vi "Test Gripper.vi"() -> ()   [LabVIEW 2018]
uses:
  <vilib>/Rock Robotics/SystemInterfaces/DIO/FPGA_DIOChannel.ctl
panel:
  in  "Boolean":bool
  in  "milliseconds to wait":u32
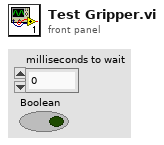
[diagram p1: front panel]
types:
  T1 = typedef "FPGA_DIOChannel.ctl" = enum8{"DIO 0", "DIO 1", "DIO 2", "DIO 3", "DIO 4", "DIO 5", "DIO 6", "DIO 7", "DIO 8", "DIO 9", "DIO MXP 0", "DIO MXP 1", "DIO MXP 2", "DIO MXP 3", "DIO MXP 4", "DIO MXP 5", "DIO MXP 6", "DIO MXP 7", "DIO MXP 8", "DIO MXP 9", "DIO MXP 10", "DIO MXP 11", "DIO MXP 12", "DIO MXP 13", "DIO MXP 14", "DIO MXP 15", "SPI Port CS1", "SPI Port CS2", "SPI Port CS3", "SPI Port MISO", "SPI Port MOSI", "Invalid"}
  T2 = typedef "WPI_DigitalOutputDevRef.ctl" = cluster{"DIO Channel":T1, "DevStatus":errorcluster}
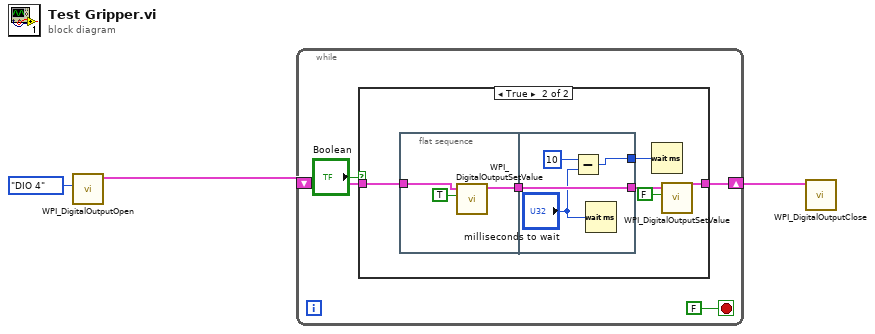
[diagram p0: block diagram]
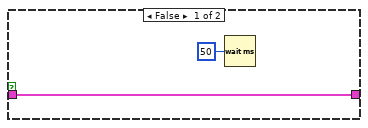
[diagram p2: hidden frame]
diagram:
  n1 = call <vilib>:"WPI_DigitalOutputOpen.vi"("DIO Channel"=FPGA_DIOChannel."DIO 4") -> ("DigitalOutputDevRef"=w1:T2)  [unwired: 9 in, 1 out]
  n2 = while {
    shift-right: [w6] -> w2
    shift-left: w1 -> [w7]
    stop <- FALSE stop-if-true
    n3 = case shown="True" "Boolean" {
      tunnel: w7 -> [w9 w13]
      tunnel: [w9 w11] -> w6
      frame False {
        n4 = Wait (ms)(milliseconds to wait=u32 50) -> ()  [unwired: 1 out]
      }
      frame True {
        n5 = flat-sequence {
          tunnel: w13 -> [w17]
          tunnel: [w16] -> w15
          tunnel: w15 -> [w22]
          tunnel: [w22] -> w12
          tunnel: [w19] -> w10
          frame #0 {
            n6 = call <vilib>:"WPI_DigitalOutputSetValue.vi"("Value"=TRUE, "DigitalOutputDevRef"=w17) -> ("DigitalOutputDevRef"=w16:T2)  [unwired: 8 in, 1 out]
          }
          frame #1 {
            n7 = Subtract(x=u32 10, y="milliseconds to wait") -> (x-y=w19:u32)
            n8 = Wait (ms)(milliseconds to wait="milliseconds to wait") -> ()  [unwired: 1 out]
          }
        }
        n9 = Wait (ms)(milliseconds to wait=w10) -> ()  [unwired: 1 out]
        n10 = call <vilib>:"WPI_DigitalOutputSetValue.vi"("Value"=FALSE, "DigitalOutputDevRef"=w12) -> ("DigitalOutputDevRef"=w11:T2)  [unwired: 8 in, 1 out]
      }
    }
  }
  n11 = call <vilib>:"WPI_DigitalOutputClose.vi"("DigitalOutputDevRef"=w2) -> ()  [unwired: 10 in, 1 out]
